vi "G#Interface_InterfaceToSpecificClass.vi"(2 "interface reference in":refnum<class "G#Object.lvclass">, 4 "error in (no error)":errorcluster, 12 "target class":refnum<class "G#Object.lvclass">) -> (22 "reference out":refnum<class "G#Object.lvclass">, 24 "error out":errorcluster)   [LabVIEW 2017, in "G#Object.lvclass"]
doc: "Cast a G#Interface reference to specified G#Object reference."
uses:
  <vilib>/addons/_AddQ/G#Object/G#Object.lvclass
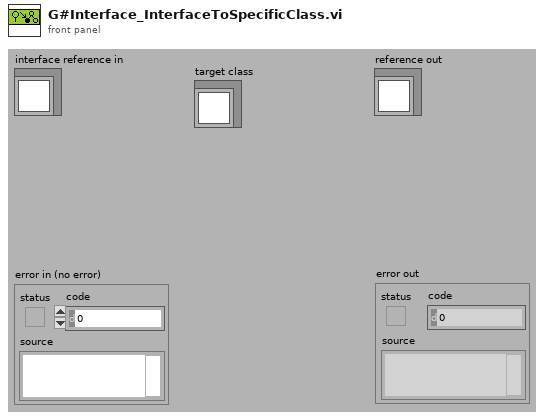
[diagram p1: front panel]
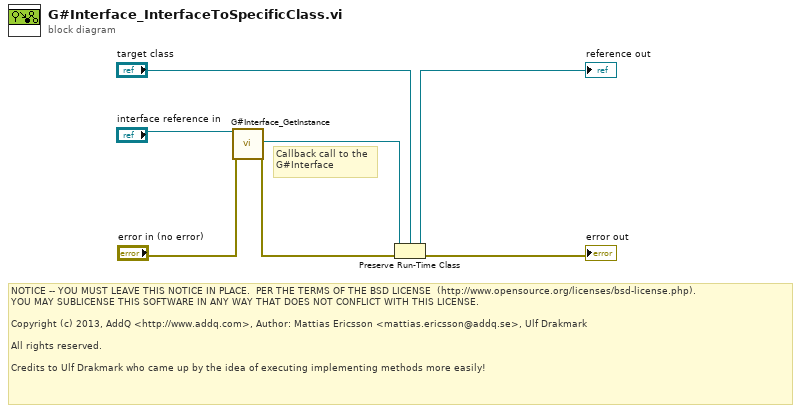
[diagram p0: block diagram]
diagram:
  # "Callback call to the\nG#Interface"
  # "NOTICE -- YOU MUST LEAVE THIS NOTICE IN PLACE.  PER THE TERMS OF THE BSD LICENSE  (http://www.opensource.org/licenses/bsd-license.php).\nYOU MAY SUBLICENSE THIS SOFTWARE IN ANY WAY THAT DOES NOT CONFLICT WITH THIS LICENSE.\n\nCopyright (c) 2013, AddQ <http://www.addq.com>, Author: Mattias Ericsson <mattias.ericsson@addq.se>, Ulf Drakmark\n\nAll rights reserved.\n\nCredits to Ulf Drakmark who came up by the idea of executing implementing methods more easily!"
  n1 = call-dynamic "G#Interface_GetInstance.vi"("reference in"="interface reference in", "error in (no error)"="error in (no error)") -> ("G#Object"=w3:refnum<class "G#Object.lvclass">, "error out"=w5:errorcluster)  [unwired: 14 in, 2 out]
  n2 = Preserve Run-Time Class(object in=w3, error in=w5, 2:"target class") -> (object out=→"reference out":refnum<class "G#Object.lvclass">, error out=→"error out":errorcluster)
